vi "OTP - Read measured cap data.vi"(5 "Frequency (MHz)":dbl=837.0, 7 "Package number":string="08", 8 "Equipment":enum16{"VNA", "LCR"}(ring), 9 "Manual Register 2 & 3 (hex)":string[][](array[string])=[["0", "0"], ["7F", "7F"], ["1", "0"], ["2", "0"], ["4", "0"], ["8", "0"], ["10", "0"], ["20", "0"], ["40", "0"], ["0", "1"], ["0", "2"], ["0", "4"], ["0", "8"], ["0", "10"], ["0", "20"], ["0", "40"]], 10 "Manual reg 2&3?":bool, 11 "file (use dialog)":path) -> (0 "Cmin (fF)":dbl, 1 "dCap (fF)":dbl[](array[numeric]), 2 "Cap (pF)":dbl[](array[numeric]), 3 "Register 2 & 3 (hex)":string[][](array[string]), 4 "Cmax (fF)":dbl)   [LabVIEW 2020]
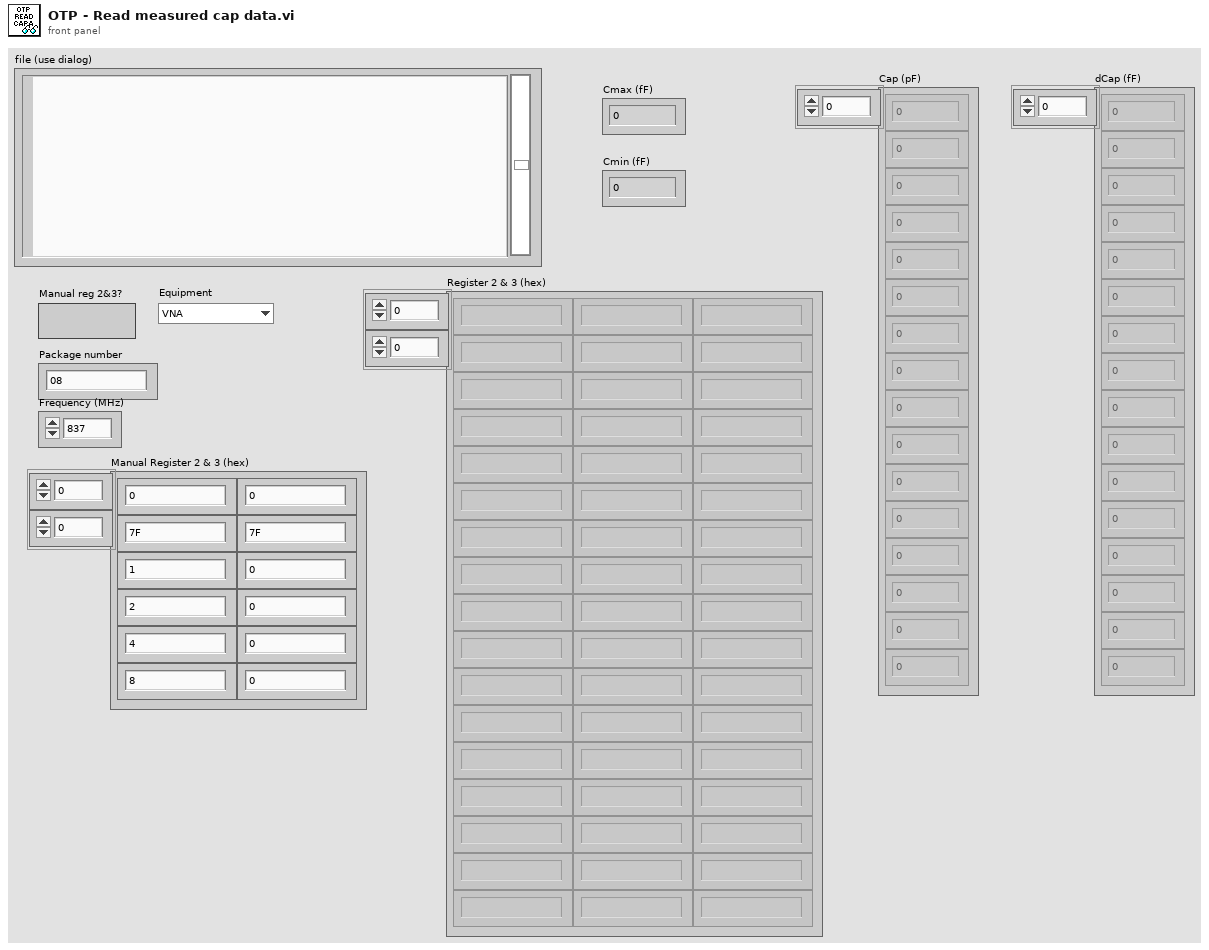
[diagram p1: front panel]
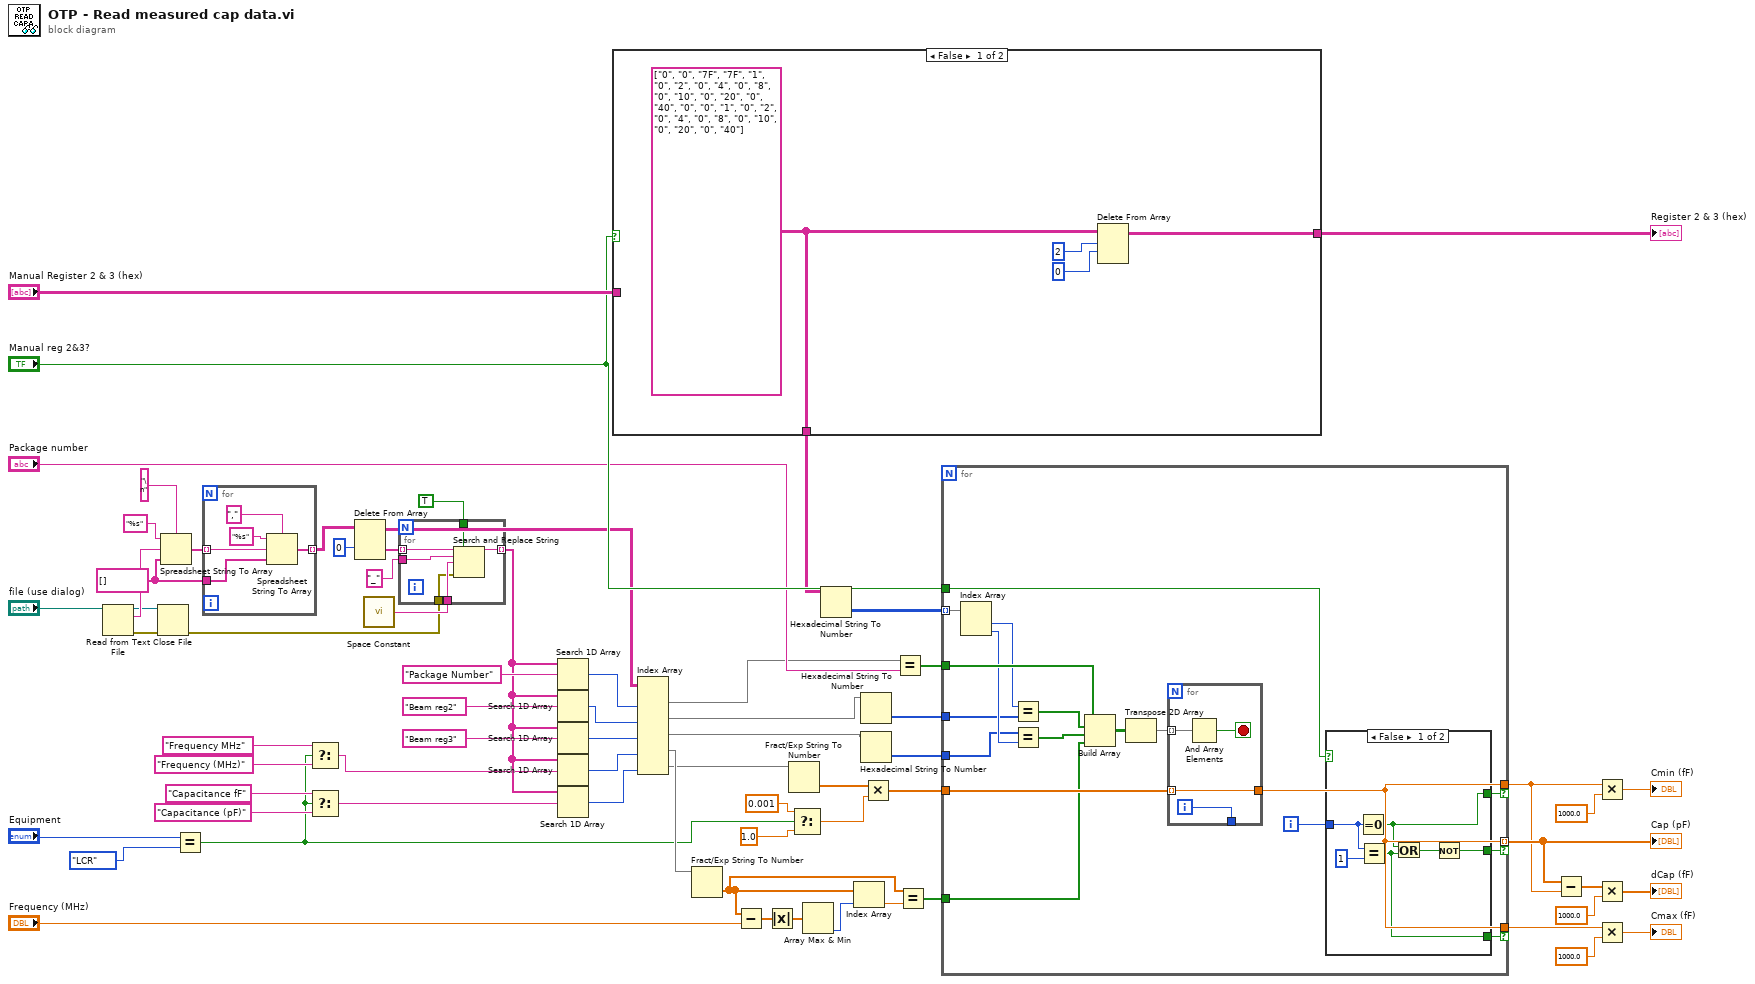
[diagram p0: block diagram]
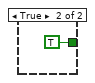
[diagram p3: hidden frame]
diagram:
  w67 = string[] []
  n1 = Read from Text File(file (use dialog)="file (use dialog)") -> (refnum out=w31:refnum<file>, text=w65:string, error out=w30:errorcluster)  [unwired: 3 in, 1 out]
  n2 = Close File(refnum=w31, error in=w30) -> (error out=w17:errorcluster)  [unwired: 1 out]
  n3 = Spreadsheet String To Array(delimiter (Tab)="\n", format string="%s", spreadsheet string=w65, array type (2D Dbl)=w67) -> (array=w68:string[])
  n4 = Equal?(x="Equipment", y=enum16{"VNA", "LCR"}."LCR") -> (x = y?=w1:bool)
  n5 = for {
    tunnel: w68 -> [w71] mode=indexing
    tunnel: w67 -> [w74]
    tunnel: [w73] -> w61 mode=indexing
    n6 = Spreadsheet String To Array(delimiter (Tab)=",", format string="%s", spreadsheet string=w71, array type (2D Dbl)=w74) -> (array=w73:string[])
  }
  n7 = Select(t="Frequency MHz" ("String 3"), s=w1, f="Frequency (MHz)" ("String 3")) -> (s? t:f=w13:string)
  n8 = Select(t="Capacitance fF" ("String 4"), s=w1, f="Capacitance (pF)" ("String 4")) -> (s? t:f=w8:string)
  n9 = Delete From Array(array=w61, index (row)=0) -> (deleted portion=w21:string[], array with subset deleted=w35:string[][])  [unwired: 2 in]
  n10 = call <vilib>:"Space Constant.vi"() -> ("String"=w18:string)
  n11 = for {
    tunnel: w21 -> [w81] mode=indexing
    tunnel: "_" ("search string") -> [w80]
    tunnel: TRUE ("replace all? (F)") -> [w79]
    tunnel: w18 -> [w78]
    tunnel: w17 -> [w77]
    tunnel: [w76] -> w16 mode=indexing
    n12 = Search and Replace String(replace all?=w79, input string=w81, search string=w80, replace string=w78, error in=w77) -> (result string=w76:string)  [unwired: 3 in, 3 out]
  }
  n13 = Search 1D Array(1D array=w16, element="Package Number" ("String")) -> (index of element=w56:i32)  [unwired: 1 in]
  n14 = Search 1D Array(1D array=w16, element="Beam reg2" ("String")) -> (index of element=w60:i32)  [unwired: 1 in]
  n15 = Search 1D Array(1D array=w16, element="Beam reg3" ("String 2")) -> (index of element=w59:i32)  [unwired: 1 in]
  n16 = Search 1D Array(1D array=w16, element=w13) -> (index of element=w58:i32)  [unwired: 1 in]
  n17 = Search 1D Array(1D array=w16, element=w8) -> (index of element=w57:i32)  [unwired: 1 in]
  n18 = case shown="False" "Manual reg 2&3?" {
    tunnel: [w85 w86] -> w34
    tunnel: [w84 w86] -> w41
    tunnel: "Manual Register 2 & 3 (hex)" -> [_ w86]
    frame False {
      w85 = string[][] [["0", "0"], ["7F", "7F"], ["1", "0"], ["2", "0"], ["4", "0"], ["8", "0"], ["10", "0"], ["20", "0"], ["40", "0"], ["0", "1"], ["0", "2"], ["0", "4"], ["0", "8"], ["0", "10"], ["0", "20"], ["0", "40"]] ("Register 2 & 3 (hex)")
      n19 = Delete From Array(array=w85, length=2, index (row)=0) -> (array with subset deleted=w84:string[][])  [unwired: 1 in, 1 out]
    }
    frame True {
    }
  }
  "Register 2 & 3 (hex)" <- w41
  n20 = Index Array(array=w35, index (col) #1=w56, index (col) #2=w60, index (col) #3=w59, index (col) #4=w58, index (col) #5=w57) -> (element #1=w28:string[], element #2=w33:string[], element #3=w32:string[], element #4=w49:string[], element #5=w7:string[])  [unwired: 5 in]
  n21 = Fract/Exp String To Number(string=w49) -> (number=w46:dbl[])  [unwired: 3 in, 1 out]
  n22 = Subtract(x=w46, y="Frequency (MHz)") -> (x-y=w48:dbl[])
  n23 = Absolute Value(x=w48) -> (abs(x)=w47:dbl[])
  n24 = Fract/Exp String To Number(string=w7) -> (number=w6:dbl[])  [unwired: 3 in, 1 out]
  n25 = Select(t=0.001, s=w1, f=1.0) -> (s? t:f=w2:dbl)
  n26 = Array Max & Min(array=w47) -> (min index (indices)=w45:i32)  [unwired: 3 out]
  n27 = Hexadecimal String To Number(string=w34) -> (number=w22:u32[][])  [unwired: 2 in, 1 out]
  n28 = Index Array(array=w46, index=w45) -> (element=w26:dbl)
  n29 = Hexadecimal String To Number(string=w33) -> (number=w24:u32[])  [unwired: 2 in, 1 out]
  n30 = Hexadecimal String To Number(string=w32) -> (number=w23:u32[])  [unwired: 2 in, 1 out]
  n31 = Multiply(x=w6, y=w2) -> (x*y=w5:dbl[])
  n32 = Equal?(x=w28, y="Package number") -> (x = y?=w27:bool[])
  n33 = Equal?(x=w46, y=w26) -> (x = y?=w25:bool[])
  n34 = for {
    tunnel: w5 -> [w104]
    tunnel: [w87] -> w54 mode=indexing if=w103
    tunnel: [w87] -> w43 if=w101
    tunnel: [w87] -> w38 if=w100
    tunnel: "Manual reg 2&3?" -> [w99]
    tunnel: w27 -> [w97]
    tunnel: w25 -> [w96]
    tunnel: w24 -> [w93]
    tunnel: w23 -> [w92]
    tunnel: w22 -> [w91] mode=indexing
    i -> [w102]
    n35 = Index Array(array=w91) -> (element #1=w94:u32, element #2=w95:u32)  [unwired: 2 in]
    n36 = Equal?(x=w94, y=w93) -> (x = y?=w90:bool[])
    n37 = Equal?(x=w92, y=w95) -> (x = y?=w89:bool[])
    n38 = Build Array(w97, w90, w89, w96) -> (w98:bool[][])
    n39 = Transpose 2D Array(2D array=w98) -> (transposed array=w88:bool[][])
    n40 = for {
      tunnel: [w115] -> w87
      tunnel: w104 -> [w115] mode=indexing
      tunnel: w88 -> [w114] mode=indexing
      tunnel: [w112] -> _
      i -> [w112]
      stop <- w113 stop-if-true
      n41 = And Array Elements(Boolean array=w114) -> (logical AND=w113:bool)
    }
    n42 = case shown="False" w99 {
      tunnel: [w110 TRUE] -> w103
      tunnel: w102 -> [w109 _]
      tunnel: [w107 _] -> w101
      tunnel: [w106 _] -> w100
      frame False {
        n43 = Equal To 0?(x=w109) -> (x = 0?=w107:bool)
        n44 = Equal?(x=w109, y=1) -> (x = y?=w106:bool)
        n45 = Or(x=w107, y=w106) -> (x .or. y?=w108:bool)
        n46 = Not(x=w108) -> (.not. x?=w110:bool)
      }
      frame True {
      }
    }
  }
  "Cap (pF)" <- w54
  n47 = Subtract(x=w54, y=w43) -> (x-y=w53:dbl[])
  n48 = Multiply(x=w43, y=1000.0) -> (x*y=→"Cmin (fF)":dbl)
  n49 = Multiply(x=w53, y=1000.0) -> (x*y=→"dCap (fF)":dbl[])
  n50 = Multiply(x=w38, y=1000.0) -> (x*y=→"Cmax (fF)":dbl)
